vi "Floats32 to bytearr.vi"(9 "bytes in":u8[](array[numeric]), 11 "Array in":sgl[](array[numeric])) -> (1 "bytes out":u8[](array[numeric]), 3 "bindata descr":T1)   [LabVIEW 2018, in "LV-Julia_ZMQ-Roundtrip_lib.lvlib"]
uses:
  LV-Julia_ZMQ-Roundtrip_lib.lvlib
panel:
  out "start":i32
  out "numtype":string
  out "length":i32
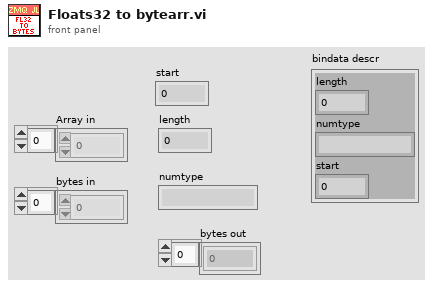
[diagram p1: front panel]
types:
  T1 = cluster{"length":i32, "numtype":string, "start":i32}
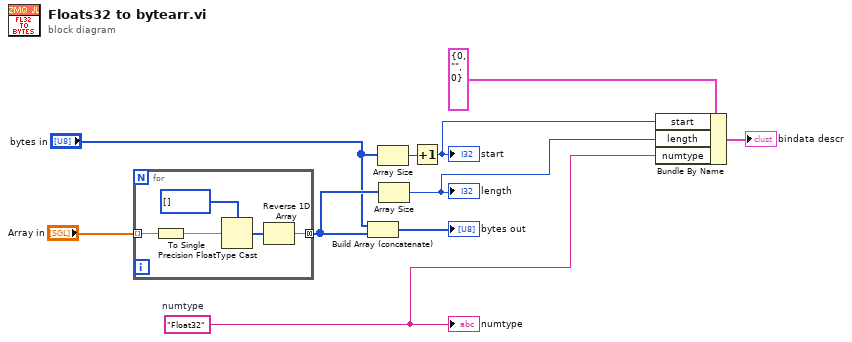
[diagram p0: block diagram]
diagram:
  w1 = "Float32"  # numtype
  n1 = for {
    tunnel: "Array in" -> [w15] mode=indexing
    tunnel: [w12] -> w9 mode=concatenating
    n2 = To Single Precision Float(number=w15) -> (single precision float=w11:sgl)
    n3 = Type Cast(type=u8[] [], x=w11) -> (*(type *) &x=w13:u8[])
    n4 = Reverse 1D Array(array=w13) -> (reversed array=w12:u8[])
  }
  n5 = Build Array (concatenate)("bytes in", w9) -> (→"bytes out":u8[])
  n6 = Array Size(array="bytes in") -> (size(s)=w7:i32)
  n7 = Array Size(array=w9) -> (size(s)=w2:i32)
  "length" <- w2
  n8 = Increment(x=w7) -> (x+1=w3:i32)
  "start" <- w3
  n9 = Bundle By Name(cluster=T1 {"length"=0, "numtype"="", "start"=0} ("bindata descr"), "start"=w3, "length"=w2, "numtype"=w1) -> (→"bindata descr":T1)
  "numtype" <- w1
